vi "Open_Argus.vi"() -> ()   [LabVIEW 2017]
panel:
  in  "remote port or service name":u16
  in  "address":string
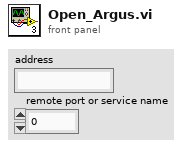
[diagram p1: front panel]
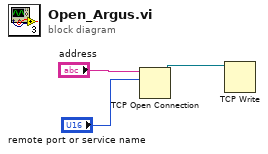
[diagram p0: block diagram]
diagram:
  n1 = TCP Open Connection(address="address", remote port or service name="remote port or service name") -> (connection ID=w1:refnum<k5>)  [unwired: 3 in, 1 out]
  n2 = TCP Write(connection ID=w1) -> ()  [unwired: 3 in, 3 out]
